vi "Raman Live Tool Set v10.1.0.vi"(1 "Exit":bool, 2 "LiveData":dbl[][](array[numeric]), 3 "RemoteIndicator":bool) -> ()   [LabVIEW 2010]
uses:
  subvi/_TypeDefs/MapFunctions.ctl
  <vilib>/Utility/miscctls.llb/LVPointTypeDef.ctl
  <vilib>/Utility/miscctls.llb/LVStringsAndValuesArrayTypeDef.ctl
  <vilib>/Utility/inputDevices.llb/closeKeyboard.vi
  <vilib>/Utility/inputDevices.llb/keyboardAcquire.vi
  <vilib>/Utility/file.llb/Read From Spreadsheet File (DBL).vi
  <vilib>/Analysis/NI_AALBase.lvlib
panel:
  in  "MapFunction":T1 caption="Mapping function" items=["Total"=0, "Peak"=4, "Area"=2, "Value"=1, "Ratio"=3]
  in  "CreateMap":bool
  in  "SpectrumCoerce":dbl caption="Limit?"
  out "XY Full Interpol.":cluster{dbl, dbl}[](array[cluster])
  out "Axes":T2
  in  "SpectrumNoise":dbl caption="Noise?"
  in  "SpectrumX":u16(ring) caption="X"
  in  "SpectrumY":u16(ring) caption="Y"
  out "Spectrum":cluster{dbl[], dbl[]}(graph) caption="Current Spectrum"
  in  "MapKeyboard":bool
  in  "MapEditColor":bool caption="Edit Color"
  in  "MapFlipColor":bool caption="Flip Color"
  in  "MapInterpolate":bool
  in  "MapSaveData":bool
  out "Map":dbl[][](graph)
  out "LoadingSpectra":bool
  in  "SourceFile":path caption="Mapping File"
  in  "MapCursorDummy":bool
  out "XY Unique":cluster{"X Unique":dbl[], "Y Unique":dbl[]}
  out "XY Full":cluster{dbl, dbl}[](array[cluster])
  out "Intensities (2D)":dbl[][](array[numeric])
  out "Wavelengths (1D)":dbl[](array[numeric])
  out "MapColorTable":u32[](array[numeric])=[0, 196608, 393216, 589824, 786432, 983040, 1179648, 1376256, 1572864, 1769472, 1966080, 2162688, 2359296, 2555904, 2752512, 2949120, 3145728, 3342336, 3538944, 3735552, 3932160, 4128768, 4325376, 4521984, 4718592, 4915200, 5111808, 5308416, 5505024, 5701632, 5898240, 6094848, 6291456, 6488064, 6684672, 6881280, 7077888, 7274496, 7471104, 7667712, 7864320, 8060928, 8257536, 8454144, 8650752, 8847360, 9043968, 9240576, 9437184, 9633792, 9830400, 10027008, 10223616, 10420224, 10616832, 10813440, 11010048, 11206656, 11403264, 11599872, 11796480, 11993088, 12189696, 12386304, 12582912, 12779520, 12976128, 13172736, 13369344, 13565952, 13762560, 13959168, 14155776, 14352384, 14548992, 14745600, 14942208, 15138816, 15335424, 15532032, 15728640, 15925248, 16121856, 16318464, 16515072, 16711680, 16712448, 16713216, 16713984, 16714752, 16715520, 16716288, 16717056, 16717824, 16718592, 16719360, 16720128, 16720896, 16721664, 16722432, 16723200, 16723968, 16724736, 16725504, 16726272, 16727040, 16727808, 16728576, 16729344, 16730112, 16730880, 16731648, 16732416, 16733184, 16733952, 16734720, 16735488, 16736256, 16737024, 16737792, 16738560, 16739328, 16740096, 16740864, 16741632, 16742400, 16743168, 16743936, 16744704, 16745472, 16746240, 16747008, 16747776, 16748544, 16749312, 16750080, 16750848, 16751616, 16752384, 16753152, 16753920, 16754688, 16755456, 16756224, 16756992, 16757760, 16758528, 16759296, 16760064, 16760832, 16761600, 16762368, 16763136, 16763904, 16764672, 16765440, 16766208, 16766976, 16767744, 16768512, 16769280, 16770048, 16770816, 16771584, 16772352, 16773120, 16773888, 16774656, 16775424, 16776192, 16776960, 16776963, 16776966, 16776969, 16776972, 16776975, 16776977, 16776980, 16776983, 16776986, 16776989, 16776992, 16776995, 16776998, 16777001, 16777004, 16777007, 16777009, 16777012, 16777015, 16777018, 16777021, 16777024, 16777027, 16777030, 16777033, 16777036, 16777038, 16777041, 16777044, 16777047, 16777050, 16777053, 16777056, 16777059, 16777062, 16777065, 16777068, 16777070, 16777073, 16777076, 16777079, 16777082, 16777085, 16777088, 16777091, 16777094, 16777097, 16777100, 16777102, 16777105, 16777108, 16777111, 16777114, 16777117, 16777120, 16777123, 16777126, 16777129, 16777132, 16777134, 16777137, 16777140, 16777143, 16777146, 16777149, 16777152, 16777155, 16777158, 16777161, 16777163, 16777166, 16777169, 16777172, 16777175, 16777178, 16777181, 16777184, 16777187, 16777190, 16777193, 16777195, 16777198, 16777201, 16777204, 16777207]
  out "MapZBounds":cluster{dbl, dbl}
  out "MapData (2D)":dbl[][](array[numeric])
  # "Cursor"
  # "Map Function"
  # "Spectrum"
  # "Raman Live Tool Set"
  # "by A. Schmitz-Wunderlich, P. Candeloro"
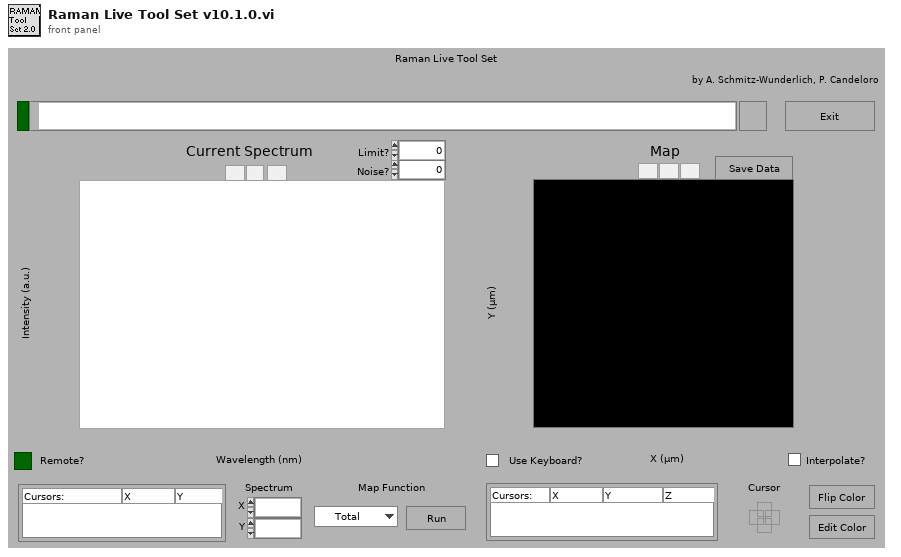
[diagram p1: front panel]
types:
  T1 = typedef "MapFunctions.ctl" = u16
  T2 = cluster{"X":cluster{"Offset":dbl, "Step Size":dbl, "Step Count":i32}, "Y":cluster{"Offset":dbl, "Step Size":dbl, "Step Count":i32}}
  T3 = typedef "LVPointTypeDef.ctl" = cluster{"Horizontal":i16, "Vertical":i16}
  T4 = enum8{"Enabled", "Disabled", "Disabled and Grayed Out"}
  T5 = enum16{"0", "1", "2", "3", "4", "5", "6", "7", "8", "9", "A", "B", "C", "D", "E", "F", "G", "H", "I", "J", "K", "L", "M", "N", "O", "P", "Q", "R", "S", "T", "U", "V", "W", "X", "Y", "Z", "F1", "F2", "F3", "F4", "F5", "F6", "F7", "F8", "F9", "F10", "F11", "F12", "F13", "F14", "F15", "ADD", "BACK", "BACKSLASH", "CAPITAL", "COMMA", "DECIMAL", "DELETE", "DIVIDE", "DOWN", "END", "EQUALS", "ESCAPE", "GRAVE (`)", "HOME", "INSERT", "LBRACKET", "LCONTROL", "LEFT", "L ALT", "LSHIFT", "LWIN", "MINUS", "MULTIPLY", "NEXT", "NUMLOCK", "NUMPAD_0", "NUMPAD_1", "NUMPAD_2", "NUMPAD_3", "NUMPAD_4", "NUMPAD_5", "NUMPAD_6", "NUMPAD_7", "NUMPAD_8", "NUMPAD_9", "PAUSE", "PERIOD", "PRIOR (PG UP)", "RBRACKET", "RCONTROL", "RETURN", "RIGHT", "R ALT", "RSHIFT", "RWIN", "SCROLL", "SEMICOLON", "SLASH", "SPACE", "SUBTRACT", "TAB", "UP", "ENTER (num pad)", "' (quote)"}
  T6 = enum16{"0", "1", "2", "3", "4", "5", "6", "7", "8", "9", "A", "B", "C", "D", "E", "F", "G", "H", "I", "J", "K", "L", "M", "N", "O", "P", "Q", "R", "S", "T", "U", "V", "W", "X", "Y", "Z", "F1", "F2", "F3", "F4", "F5", "F6", "F7", "F8", "F9", "F10", "F11", "F12", "F13", "F14", "F15", "ADD", "BACK", "BACKSLASH", "CAPITAL", "COMMA", "DECIMAL", "DELETE", "DIVIDE", "DOWN", "END", "EQUALS", "ESCAPE", "GRAVE (`)", "HOME", "INSERT", "LBRACKET", "LCONTROL", "LEFT", "L ALT", "LSHIFT", "LWIN", "MINUS", "MULTIPLY", "NEXT", "NUMLOCK", "NUMPAD_0", "NUMPAD_1", "NUMPAD_2", "NUMPAD_3", "NUMPAD_4", "NUMPAD_5", "NUMPAD_6", "NUMPAD_7", "NUMPAD_8", "NUMPAD_9", "PAUSE", "PERIOD", "PRIOR (PG UP)", "RBRACKET", "RCONTROL", "RETURN", "RIGHT", "R ALT", "RSHIFT", "RWIN", "SCROLL", "SEMICOLON", "SLASH", "SPACE", "SUBTRACT", "TAB", "UP", "ENTER (num pad)", "' (quote)"}[]
  T7 = cluster{"Name":string, "Color":u32, "Style":u8, "Point Style":u8, "Name Visible":bool, "Allow Drag":bool, "Cursor Mode":u32, "Plot":i32, "Index":i32, "Position":cluster{"X":dbl, "Y":dbl}, "X Scale":u32, "Y Scale":u32, "Watch Plots":i32[], "Watch All Plots":bool, "Plot Area":i32, "Label Offset":cluster{"X":dbl, "Y":dbl}}
  T8 = cluster{"Name":string, "Color":u32, "Style":u8, "Point Style":u8, "Name Visible":bool, "Allow Drag":bool, "Cursor Mode":u32, "Plot":i32, "Index":i32, "Position":cluster{"X":dbl, "Y":dbl}, "X Scale":u32, "Y Scale":u32, "Watch Plots":i32[], "Watch All Plots":bool, "Plot Area":i32, "Label Offset":cluster{"X":dbl, "Y":dbl}}[]
  T9 = typedef "LVCursorListTypeDef.ctl" = cluster{"Name":string, "Color":u32, "Style":u8, "Point Style":u8, "Name Visible":bool, "Allow Drag":bool, "Cursor Mode":u32, "Plot":i32, "Index":i32, "Position":cluster{"X":dbl, "Y":dbl}, "X Scale":u32, "Y Scale":u32, "Watch Plots":i32[], "Watch All Plots":bool, "Plot Area":i32, "Label Offset":cluster{"X":dbl, "Y":dbl}}[]
  T10 = typedef "LVPointDoubleTypeDef.ctl" = cluster{"Cursor X":dbl, "Cursor Y":dbl}
  T11 = typedef "LVStringsAndValuesArrayTypeDef.ctl" = cluster{"String":string, "Value":ext}[]
  T12 = enum32{"invalid app kind", "Development System", "Run Time System", "Student Edition", "Embedded LabVIEW", "Evaluation", "Custom"}
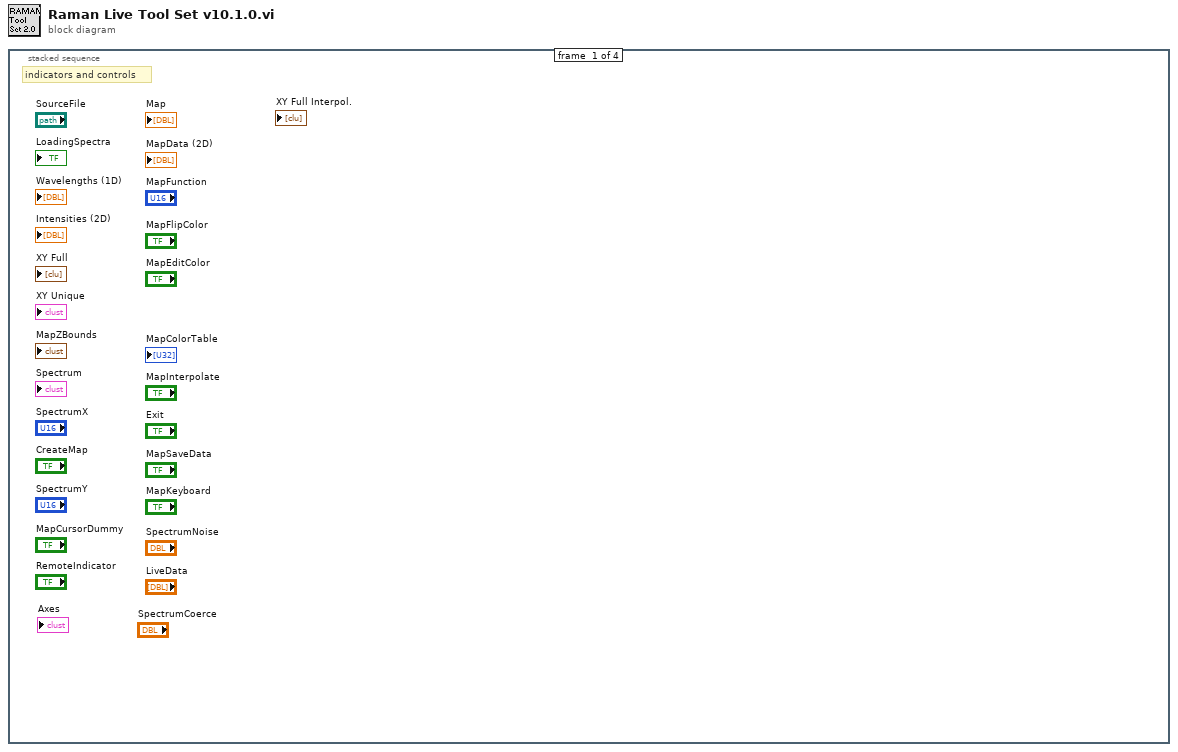
[diagram p0: block diagram]
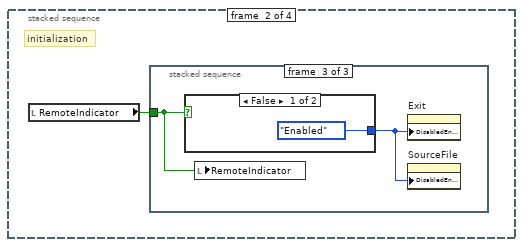
[diagram p2: hidden frame]
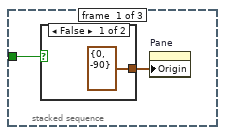
[diagram p3: hidden frame]
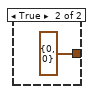
[diagram p4: hidden frame]
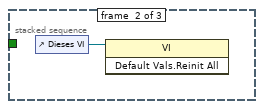
[diagram p5: hidden frame]
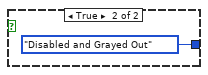
[diagram p6: hidden frame]
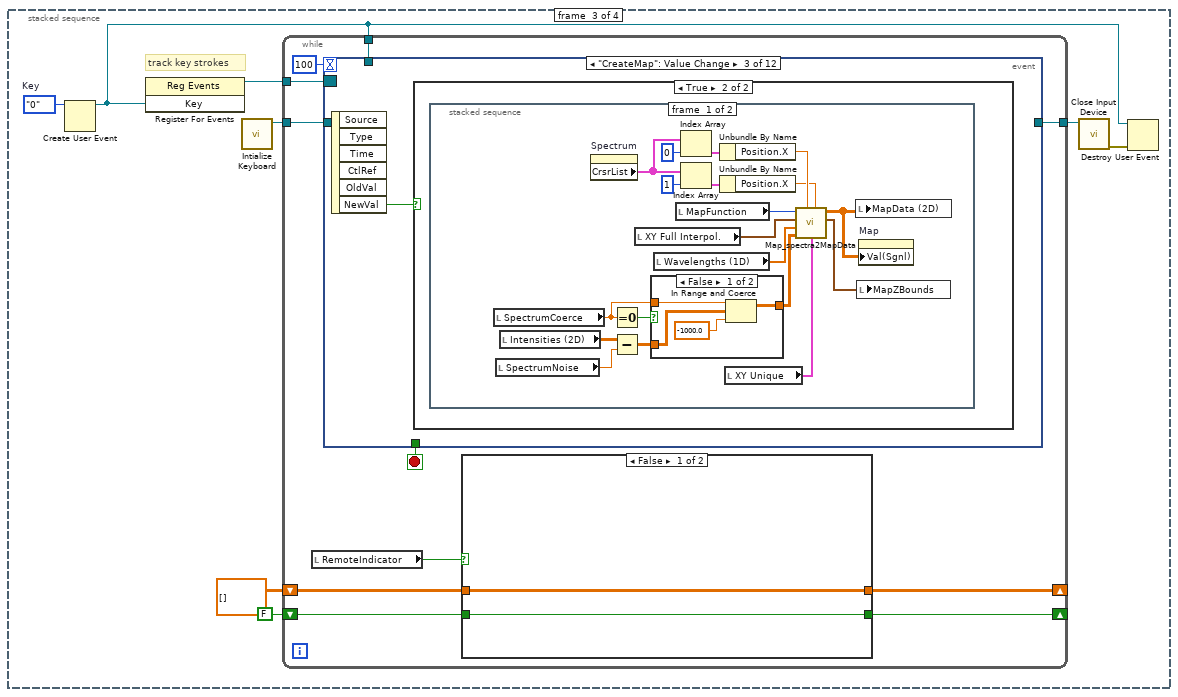
[diagram p7: hidden frame]
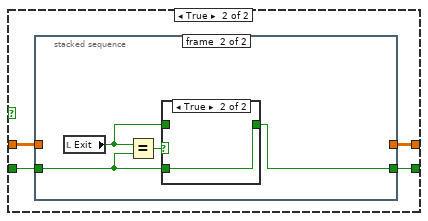
[diagram p8: hidden frame]
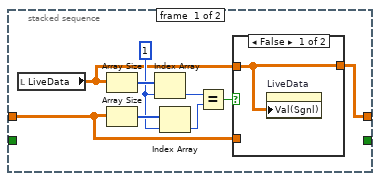
[diagram p9: hidden frame]
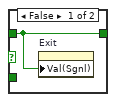
[diagram p11: hidden frame]
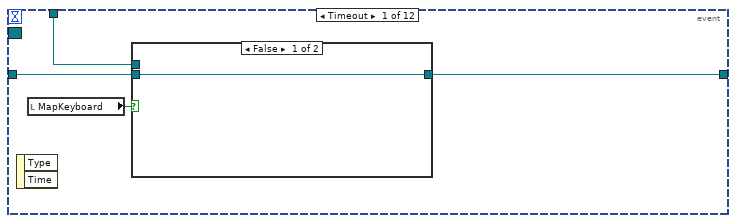
[diagram p12: hidden frame]
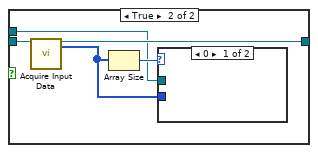
[diagram p13: hidden frame]
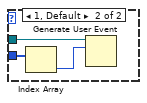
[diagram p14: hidden frame]
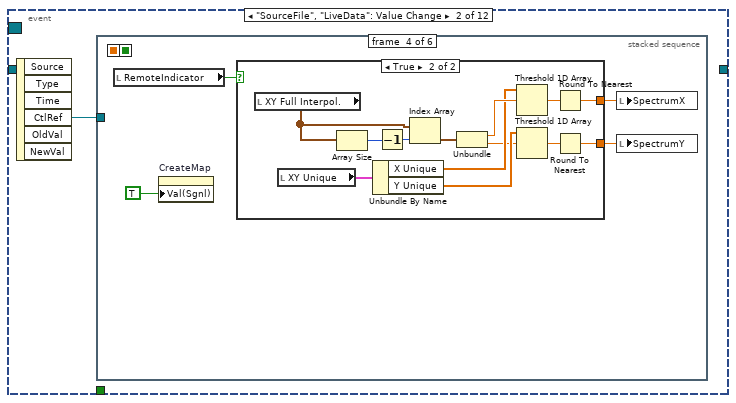
[diagram p15: hidden frame]
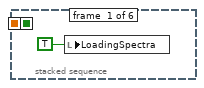
[diagram p16: hidden frame]
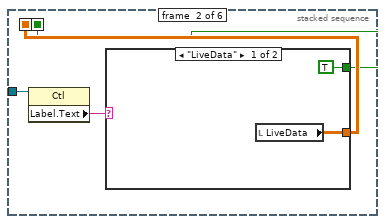
[diagram p17: hidden frame]
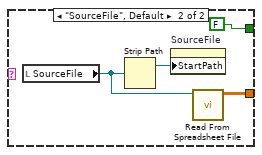
[diagram p18: hidden frame]
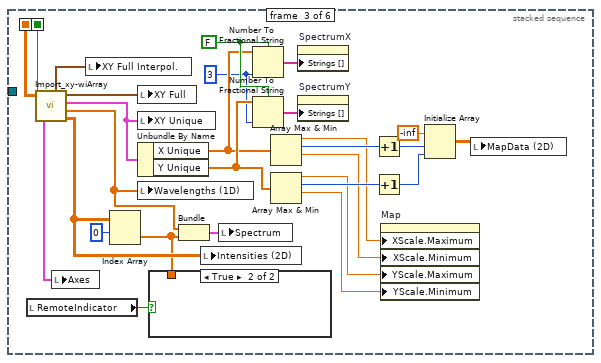
[diagram p19: hidden frame]
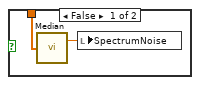
[diagram p20: hidden frame]
diagram:
  n1 = stacked-sequence {
    frame #0 {
      # "indicators and controls"
    }
    frame #1 {
      # "initialization"
      n2 = local read "RemoteIndicator"() -> (w1:bool)
      n3 = stacked-sequence {
        tunnel: w1 -> [w2 _ w7]
        frame #0 {
          n4 = case shown="False" w2 {
            tunnel: [T3 {"Horizontal"=0, "Vertical"=-90} ("Origin") T3 {"Horizontal"=0, "Vertical"=0} ("Origin")] -> w3
            frame False {
            }
            frame True {
            }
          }
          n5 = property on="Pane" class="Pane"("Origin"=w3) -> ()  [unwired: 2 in, 2 out]
        }
        frame #1 {
          n6 = control-ref of="Dieses VI"() -> (w6:refnum<vi>)
          n7 = invoke class="VI" method="Default Vals.Reinit All"(reference=w6) -> ()  [unwired: 2 in, 3 out]
        }
        frame #2 {
          n8 = case shown="False" w7 {
            tunnel: [T4."Enabled" ("Deaktiviert") T4."Disabled and Grayed Out" ("Deaktiviert")] -> w8
            frame False {
            }
            frame True {
            }
          }
          n9 = local write "RemoteIndicator"(w7) -> ()
          n10 = property on="Exit" class="Bool (strict)"("DisabledEnum"=w8) -> ()  [unwired: 2 in, 2 out]
          n11 = property on="SourceFile" class="Path"("DisabledEnum"=w8) -> ()  [unwired: 2 in, 2 out]
        }
      }
    }
    frame #2 {
      w18 = T5."0"  # Key
      # "track key strokes"
      n12 = Create User Event(user event datatype=w18) -> (user event=w15:refnum<user-event>)  [unwired: 1 in, 1 out]
      n13 = register-events(w15) -> (reference out=w16:refnum<event-registration>)  [unwired: 2 in, 1 out]
      n14 = call <vilib>:"Intialize Keyboard.vi"() -> ("device ID"=w14:refnum<k1>)  [unwired: 10 in, 1 out]
      n15 = while {
        tunnel: w16 -> [w28]
        tunnel: w15 -> [w27]
        tunnel: w14 -> [w26]
        tunnel: [w25] -> w13
        shift-right: [w21] -> _
        shift-left: dbl[][] [] ("LiveData") -> [w22]
        shift-right: [w19] -> _
        shift-left: FALSE -> [w20]
        stop <- w29 stop-if-true
        n16 = local read "RemoteIndicator"() -> (w23:bool)
        n17 = event shown="[2] \"CreateMap\": Value Change" {
          selector: w28 -> [_ _ _ _ _ _ _ _ _ _ _ _]
          dyn-events: _ -> [_ _ _ _ _ _ _ _ _ _ _ _]
          timeout: 100 -> [_ _ _ _ _ _ _ _ _ _ _ _]
          tunnel: [_ _ _ _ _ _ _ _ _ _ _ w329] -> w29
          tunnel: w27 -> [w56 _ _ _ _ _ _ _ _ _ _ _]
          tunnel: w26 -> [w55 _ _ _ _ _ _ _ _ _ _ _]
          tunnel: [w53 _ _ _ _ _ _ _ _ _ _ _] -> w25
          event Timeout {
            n18 = event-data() -> ()  [unwired: 1 in, 2 out]
            n19 = local read "MapKeyboard"() -> (w54:bool)
            n20 = case shown="False" w54 {
              tunnel: [w57 w62] -> w53
              tunnel: w56 -> [_ w59]
              tunnel: w55 -> [w57 w58]
              frame False {
              }
              frame True {
                n21 = call-poly <vilib>:"Acquire Input Data.vi"("device ID"=w58) -> ("device ID"=w62:refnum<k1>, "keys pressed"=w61:T6)  [unwired: 16 in, 1 out]
                n22 = Array Size(array=w61) -> (size(s)=w60:i32)
                n23 = case shown="0" w60 {
                  tunnel: w59 -> [_ w65]
                  tunnel: w61 -> [_ w63]
                  frame 0 {
                  }
                  frame 1, Default {
                    n24 = Index Array(array=w63) -> (element=w64:T5)  [unwired: 1 in]
                    n25 = Generate User Event(user event=w65, event data cluster=w64) -> ()  [unwired: 1 in, 2 out]
                  }
                }
              }
            }
          }
          event "SourceFile", "LiveData": Value Change {
            n26 = event-data() -> ("CtlRef"=w66:refnum<vi>)  [unwired: 1 in, 5 out]
            n27 = stacked-sequence {
              seq-local: [_ w69 _ _ _ _] -> [_ _ w87 _ _ _]
              seq-local: [_ w68 _ _ _ _] -> [_ _ w80 _ _ _]
              tunnel: w66 -> [_ w71 _ _ _ _]
              frame #0 {
                n28 = local write "LoadingSpectra"(TRUE ("Loading\nSpectra")) -> ()
              }
              frame #1 {
                n29 = property class="Ctl"(reference=w71) -> ("Label.Text"=w70:string)  [unwired: 1 in, 2 out]
                n30 = case shown="\"LiveData\"" w70 {
                  tunnel: [w73 w75] -> w69
                  tunnel: [TRUE FALSE] -> w68
                  frame "LiveData" {
                    n31 = local read "LiveData"() -> (w73:dbl[][])
                  }
                  frame "SourceFile", Default {
                    n32 = local read "SourceFile"() -> (w76:path)
                    n33 = Strip Path(path=w76) -> (stripped path=w77:path)  [unwired: 1 out]
                    n34 = property on="SourceFile" class="Path"("StartPath"=w77) -> ()  [unwired: 2 in, 2 out]
                    n35 = call-poly <vilib>:"Read From Spreadsheet File.vi"("file path (dialog if empty)"=w76) -> ("all rows"=w75:dbl[][])  [unwired: 6 in, 4 out]
                  }
                }
              }
              frame #2 {
                w94 = i16 3 ("Genauigkeit (6)")
                w101 = FALSE ("Systemdezimalzeichen verwenden (T)")
                n36 = local read "RemoteIndicator"() -> (w81:bool)
                n37 = call "Import_xy-wiArray.vi"("InputArray"=w87, "Uniform"=w80) -> ("XY Full"=w79:cluster{dbl, dbl}[], "XY Unique"=w84:cluster{"X Unique":dbl[], "Y Unique":dbl[]}, "Wavelength"=w85:dbl[], "Intensity"=w86:dbl[][], "XY Full Interpol."=w78:cluster{dbl, dbl}[], "Axes"=w82:T2)
                n38 = local write "Axes"(w82) -> ()
                n39 = local write "XY Full Interpol."(w78) -> ()
                n40 = Index Array(array=w86, index (row)=0 ("Index (Zeile)")) -> (element=w83:dbl[])  [unwired: 1 in]
                n41 = local write "XY Full"(w79) -> ()
                n42 = local write "XY Unique"(w84) -> ()
                n43 = Unbundle By Name(w84) -> ("X Unique"=w95:dbl[], "Y Unique"=w96:dbl[])
                n44 = local write "Wavelengths (1D)"(w85) -> ()
                n45 = case shown="True" w81 {
                  tunnel: w83 -> [w106 _]
                  frame False {
                    n46 = call <vilib>:"Median.vi"("X"=w106) -> ("median"=w107:dbl)  [unwired: 1 out]
                    n47 = local write "SpectrumNoise"(w107) -> ()
                  }
                  frame True {
                  }
                }
                n48 = Bundle("Wavelength"=w85, "Intensity"=w83) -> (w105:cluster{"Wavelength":dbl[], "Intensity":dbl[]})  [unwired: 1 in]
                n49 = local write "Intensities (2D)"(w86) -> ()
                n50 = local write "Spectrum"(w105) -> ()
                n51 = Number To Fractional String(use system decimal point (T)=w101, number=w95, precision (6)=w94) -> (F-format string=w98:string[])  [unwired: 1 in]
                n52 = Number To Fractional String(use system decimal point (T)=w101, number=w96, precision (6)=w94) -> (F-format string=w97:string[])  [unwired: 1 in]
                n53 = Array Max & Min(array=w95) -> (max value=w91:dbl, max index (indices)=w93:i32, min value=w90:dbl)  [unwired: 1 out]
                n54 = Array Max & Min(array=w96) -> (max value=w89:dbl, max index (indices)=w92:i32, min value=w88:dbl)  [unwired: 1 out]
                n55 = property on="SpectrumX" class="Ring (strict)"("Strings []"=w98) -> ()  [unwired: 2 in, 2 out]
                n56 = property on="SpectrumY" class="Ring (strict)"("Strings []"=w97) -> ()  [unwired: 2 in, 2 out]
                n57 = Increment(x=w93) -> (x+1=w102:i32)
                n58 = Increment(x=w92) -> (x+1=w103:i32)
                n59 = property on="Map" class="IntGraph (strict)"("XScale.Maximum"=w91, "XScale.Minimum"=w90, "YScale.Maximum"=w89, "YScale.Minimum"=w88) -> ()  [unwired: 2 in, 2 out]
                n60 = Initialize Array(-inf, w102, w103) -> (w100:dbl[][])
                n61 = local write "MapData (2D)"(w100) -> ()
              }
              frame #3 {
                n62 = local read "RemoteIndicator"() -> (w111:bool)
                n63 = property on="CreateMap" class="Bool (strict)"("Val(Sgnl)"=TRUE ("Wert (signalisierend)")) -> ()  [unwired: 2 in, 2 out]
                n64 = case shown="True" w111 {
                  tunnel: [w112 w113] -> w110
                  tunnel: [w112 w114] -> w109
                  frame False {
                    w112 = 0
                  }
                  frame True {
                    n65 = local read "XY Full Interpol."() -> (w122:cluster{dbl, dbl}[])
                    n66 = local read "XY Unique"() -> (w125:cluster{"X Unique":dbl[], "Y Unique":dbl[]})
                    n67 = Array Size(array=w122) -> (size(s)=w124:i32)
                    n68 = Unbundle By Name(w125) -> ("X Unique"=w118:dbl[], "Y Unique"=w117:dbl[])
                    n69 = Decrement(x=w124) -> (x-1=w123:i32)
                    n70 = Index Array(array=w122, index=w123) -> (element=w121:cluster{dbl, dbl})
                    n71 = Unbundle(w121) -> (w119:dbl, w116:dbl)
                    n72 = Threshold 1D Array(2:w119, 3:w118) -> (0:w120:dbl)  [unwired: 1 in]
                    n73 = Threshold 1D Array(2:w116, 3:w117) -> (0:w115:dbl)  [unwired: 1 in]
                    n74 = Round To Nearest(number=w120) -> (nearest integer value=w113:dbl)
                    n75 = Round To Nearest(number=w115) -> (nearest integer value=w114:dbl)
                  }
                }
                n76 = local write "SpectrumX"(w110) -> ()
                n77 = local write "SpectrumY"(w109) -> ()
              }
              frame #4 {
                w135 = i8 2 ("y")
                w143 = T7 {"Name"="cursor", "Color"=1985280, "Style"=2, "Point Style"=6, "Name Visible"=FALSE, "Allow Drag"=TRUE, "Cursor Mode"=0, "Plot"=0, "Index"=0, "Position"={"X"=0.0, "Y"=0.0}, "X Scale"=0, "Y Scale"=0, "Watch Plots"=[], "Watch All Plots"=FALSE, "Plot Area"=0, "Label Offset"={"X"=0.0, "Y"=0.0}}  # cursorConst
                n78 = local read "Axes"() -> (w139:T2)
                n79 = Unbundle By Name(w139) -> ("X.Offset"=w138:dbl, "X.Step Size"=w137:dbl, "Y.Offset"=w134:dbl, "Y.Step Size"=w136:dbl)
                n80 = Divide(x=w137, y=w135) -> (x/y=w133:dbl)
                n81 = Divide(x=w136, y=w135) -> (x/y=w132:dbl)
                n82 = Add(x=w138, y=w133) -> (x+y=w130:dbl)
                n83 = Add(x=w134, y=w132) -> (x+y=w131:dbl)
                n84 = Bundle(w130, w131) -> (w128:cluster{dbl, dbl})  [unwired: 1 in]
                n85 = Bundle By Name(cluster=w143, "Name"="Spot", "Cursor Mode"=u32 0, "Position"=w128) -> (w127:T7)
                n86 = Build Array(w127) -> (w126:T8)
                n87 = property on="Map" class="IntGraph (strict)"("CrsrLis"=w126, "Cursor.Cursor Style"=u8 8, "Cursor.Cursor Point Style"=u8 5, "Cursor.Cursor Color"=u32 16448250 ("Color")) -> ()  [unwired: 2 in, 2 out]
              }
              frame #5 {
                n88 = local write "LoadingSpectra"(FALSE ("Loading\nSpectra")) -> ()
              }
            }
          }
          event "CreateMap": Value Change {
            n89 = event-data() -> ("NewVal"=w146:bool)  [unwired: 1 in, 5 out]
            n90 = case shown="True" w146 {
              frame False {
              }
              frame True {
                n91 = stacked-sequence {
                  frame #0 {
                    n92 = local read "SpectrumCoerce"() -> (w151:dbl)
                    n93 = local read "SpectrumNoise"() -> (w154:dbl)
                    n94 = local read "Intensities (2D)"() -> (w147:dbl[][])
                    n95 = property on="Spectrum" class="XYGraph (strict)"() -> ("CrsrList"=w158:T9)  [unwired: 2 in, 2 out]
                    n96 = Equal To 0?(x=w151) -> (x = 0?=w150:bool)
                    n97 = Subtract(x=w147, y=w154) -> (x-y=w148:dbl[][])
                    n98 = local read "XY Full Interpol."() -> (w153:cluster{dbl, dbl}[])
                    n99 = case shown="False" w150 {
                      tunnel: w151 -> [w169 _]
                      tunnel: [w168 w170] -> w149
                      tunnel: w148 -> [w167 w170]
                      frame False {
                        n100 = In Range and Coerce(upper limit=w169, x=w167, lower limit=-1000.0 ("SpectrumCoerce")) -> (coerced(x)=w168:dbl[][])  [unwired: 1 out]
                      }
                      frame True {
                      }
                    }
                    n101 = local read "Wavelengths (1D)"() -> (w165:dbl[])
                    n102 = local read "MapFunction"() -> (w155:T1)
                    n103 = Index Array(array=w158, index=0 ("Index")) -> (element=w161:T7)
                    n104 = Index Array(array=w158, index=1 ("Index")) -> (element=w162:T7)
                    n105 = Unbundle By Name(w161) -> ("Position.X"=w157:dbl)
                    n106 = Unbundle By Name(w162) -> ("Position.X"=w156:dbl)
                    n107 = local read "XY Unique"() -> (w152:cluster{"X Unique":dbl[], "Y Unique":dbl[]})
                    n108 = call "Map_spectra2MapData.vi"("Intensity"=w149, "Wavelength"=w165, "XY Unique"=w152, "XY Full"=w153, "MapFunction"=w155, "X1"=w157, "X2"=w156) -> ("MapZBounds"=w163:cluster{sgl, sgl}, "MapData"=w164:sgl[][])  [unwired: 2 in]
                    n109 = local write "MapData (2D)"(w164) -> ()
                    n110 = local write "MapZBounds"(w163) -> ()
                    n111 = property on="Map" class="IntGraph (strict)"("Val(Sgnl)"=w164) -> ()  [unwired: 2 in, 2 out]
                  }
                  frame #1 {
                    n112 = local read "SpectrumX"() -> (w172:u16)
                    n113 = local write "CreateMap"(FALSE ("Value")) -> ()
                    n114 = property on="SpectrumX" class="Ring (strict)"("Val(Sgnl)"=w172) -> ()  [unwired: 2 in, 2 out]
                  }
                }
              }
            }
          }
          event "Map", "MapInterpolate", "MapFlipColor": Value Change {
            n115 = event-data() -> ()  [unwired: 1 in, 6 out]
            n116 = stacked-sequence {
              seq-local: [w173 _ _ _ _] -> [_ _ w198 _ _]
              frame #0 {
                n117 = local read "MapInterpolate"() -> (w178:bool)
                n118 = local read "MapData (2D)"() -> (w177:dbl[][])
                n119 = local read "XY Unique"() -> (w174:cluster{"X Unique":dbl[], "Y Unique":dbl[]})
                n120 = local read "Axes"() -> (w176:T2)
                n121 = case shown="True" w178 {
                  tunnel: [w180 w184] -> w175
                  tunnel: w177 -> [w180 w185]
                  tunnel: w176 -> [w179 _]
                  tunnel: w174 -> [_ w182]
                  tunnel: [w179 w181] -> w173
                  frame False {
                  }
                  frame True {
                    n122 = call "Map_interpolateXYZ.vi"("Level"=3, "MapData (2D)"=w185, "XY Unique"=w182) -> ("Z Interpoliert"=w184:dbl[][], "Axes"=w181:T2)  [unwired: 1 out]
                  }
                }
                n123 = local write "Map"(w175) -> ()
              }
              frame #1 {
                w193 = u32 0 ("Color")
                n124 = local read "MapColorTable"() -> (w191:u32[])
                n125 = local read "MapZBounds"() -> (w192:cluster{dbl, dbl})
                n126 = local read "MapFlipColor"() -> (w190:bool)
                n127 = Unbundle(w192) -> (w196:dbl, w189:dbl)
                n128 = Greater Than 0?(x=w189) -> (x > 0?=w187:bool)
                n129 = Reverse 1D Array(array=w191) -> (reversed array=w195:u32[])
                n130 = Select(t=w189, s=w187, f=0.0) -> (s? t:f=w186:dbl)
                n131 = Select(t=w195, s=w190, f=w191) -> (s? t:f=w194:u32[])
                n132 = property on="Map" class="IntGraph (strict)"("ZScale.Interpolate Color"=TRUE ("Z Scale.Interpolate Color"), "ZScale.Maximum"=w196, "ZScale.Minimum"=w186, "Color Table"=w194, "ZScale.High Color"=w193, "ZScale.Low Color"=w193) -> ()  [unwired: 2 in, 2 out]
              }
              frame #2 {
                n133 = Unbundle By Name(w198) -> ("X.Offset"=w202:dbl, "X.Step Size"=w201:dbl, "Y.Offset"=w200:dbl, "Y.Step Size"=w199:dbl)
                n134 = property on="Map" class="IntGraph (strict)"("XScale.Offset"=w202, "XScale.Multiplier"=w201, "YScale.Offset"=w200, "YScale.Multiplier"=w199) -> ()  [unwired: 2 in, 2 out]
              }
              frame #3 {
                w203 = u8 1 ("X-Achse.Achsenanpassung")
                n135 = property on="Map" class="IntGraph (strict)"("XScale.ScaleFit"=w203, "YScale.ScaleFit"=w203, "ZScale.ScaleFit"=u8 0 ("Z-Achse.Achsenanpassung")) -> ()  [unwired: 2 in, 2 out]
              }
              frame #4 {
                n136 = local read "SpectrumX"() -> (w205:u16)
                n137 = property on="SpectrumX" class="Ring (strict)"("Val(Sgnl)"=w205) -> ()  [unwired: 2 in, 2 out]
              }
            }
          }
          event "MapEditColor": Value Change {
            n138 = event-data() -> ("NewVal"=w206:bool)  [unwired: 1 in, 5 out]
            n139 = case shown="True" w206 {
              frame False {
              }
              frame True {
                n140 = flat-sequence {
                  frame #0 {
                    n141 = local read "MapColorTable"() -> (w207:u32[])
                    n142 = call "MapColor_makeRamp.vi"("ColorMap\narray IN"=w207) -> ("ColorMap\narray OUT"=w208:u32[])
                    n143 = local write "MapColorTable"(w208) -> ()
                  }
                  frame #1 {
                    n144 = local read "MapData (2D)"() -> (w210:dbl[][])
                    n145 = local write "MapEditColor"(FALSE ("Value")) -> ()
                    n146 = property on="Map" class="IntGraph (strict)"("Val(Sgnl)"=w210) -> ()  [unwired: 2 in, 2 out]
                  }
                }
              }
            }
          }
          event "MapSaveData": Value Change {
            n147 = event-data() -> ("NewVal"=w211:bool)  [unwired: 1 in, 5 out]
            n148 = case shown="True" w211 {
              frame False {
              }
              frame True {
                n149 = flat-sequence {
                  frame #0 {
                    n150 = property on="MapFunction" class="Ring (strict)"() -> ("RingText.Text"=w213:string)  [unwired: 2 in, 2 out]
                    n151 = local read "SourceFile"() -> (w212:path)
                    n152 = control-ref of="Spectrum"() -> (w214:refnum<vi>)
                    n153 = call "Export_mapFileName.vi"("MapFunctionStr"=w213, "Spectrum"=w214, "SourceFile"=w212) -> ("Dateipfad"=w215:path)
                    n154 = local read "XY Full"() -> (w216:cluster{dbl, dbl}[])
                    n155 = local read "Map"() -> (w217:dbl[][])
                    n156 = call "Export_map2Text.vi"("MapData (2D)"=w217, "XY Full"=w216, "ExportPath"=w215) -> ()  [unwired: 1 in]
                  }
                  frame #1 {
                    n157 = local write "MapSaveData"(FALSE ("Value")) -> ()
                    n158 = Wait (ms)(milliseconds to wait=u32 300) -> ()  [unwired: 1 out]
                  }
                }
              }
            }
          }
          event Value Change {
            n159 = event-data() -> ()  [unwired: 1 in, 6 out]
            n160 = local read "MapFunction"() -> (w220:T1)
            n161 = control-ref of="Spectrum"() -> (w221:refnum<vi>)
            n162 = call "SpectrumCursor_init.vi"("MapFunction"=w220, "Spectrum"=w221) -> ()  [unwired: 1 in]
          }
          event "SpectrumY", "SpectrumX", "SpectrumNoise", "SpectrumCoerce": Value Change {
            n163 = event-data() -> ()  [unwired: 1 in, 6 out]
            n164 = local read "XY Unique"() -> (w239:cluster{"X Unique":dbl[], "Y Unique":dbl[]})
            n165 = local read "SpectrumX"() -> (w234:u16)
            n166 = local read "SpectrumY"() -> (w235:u16)
            n167 = Unbundle By Name(w239) -> ("X Unique"=w237:dbl[], "Y Unique"=w236:dbl[])
            n168 = local read "Intensities (2D)"() -> (w241:dbl[][])
            n169 = local read "SpectrumCoerce"() -> (w225:dbl)
            n170 = local read "XY Full Interpol."() -> (w227:cluster{dbl, dbl}[])
            n171 = local read "SpectrumNoise"() -> (w238:dbl)
            n172 = Index Array(array=w237, index=w234) -> (element=w244:dbl)
            n173 = Index Array(array=w236, index=w235) -> (element=w243:dbl)
            n174 = Bundle(cluster=cluster{dbl, dbl} {0.0, 0.0} ("Element"), w244, w243) -> (w230:cluster{dbl, dbl})
            n175 = Equal To 0?(x=w225) -> (x = 0?=w226:bool)
            n176 = property on="Map" class="IntGraph (strict)"("Cursor.Cursor Position"=w230) -> ()  [unwired: 2 in, 2 out]
            n177 = while {
              tunnel: w227 -> [w256] mode=indexing
              tunnel: w230 -> [w257]
              tunnel: [w255] -> w232
              tunnel: [w252] -> w229
              tunnel: w227 -> [w253]
              i -> [w255]
              stop <- w250 stop-if-true
              n178 = Array Size(array=w253) -> (size(s)=w254:i32)
              n179 = Equal?(x=w256, y=w257) -> (x = y?=w252:bool)
              n180 = Greater?(x=w255, y=w254) -> (0:w251:bool)
              n181 = Or(x=w251, y=w252) -> (x .or. y?=w250:bool)
            }
            n182 = local read "Wavelengths (1D)"() -> (w242:dbl[])
            n183 = Select(t=w232, s=w229, f=u8 0) -> (s? t:f=w228:i32)
            n184 = Index Array(array=w241, index (row)=w228) -> (element=w224:dbl[])  [unwired: 1 in]
            n185 = Subtract(x=w224, y=w238) -> (x-y=w223:dbl[])
            n186 = case shown="False" w226 {
              tunnel: w225 -> [w248 _]
              tunnel: w223 -> [w247 w249]
              tunnel: [w246 w249] -> w222
              frame False {
                n187 = In Range and Coerce(upper limit=w248, x=w247, lower limit=-1000.0 ("SpectrumCoerce")) -> (coerced(x)=w246:dbl[])  [unwired: 1 out]
              }
              frame True {
              }
            }
            n188 = Bundle("Wavelengths (1D)"=w242, w222) -> (w240:cluster{"Wavelengths (1D)":dbl[], dbl[]})  [unwired: 1 in]
            n189 = local write "Spectrum"(w240) -> ()
          }
          event "Map": Cursor Release; "MapCursorDummy": Value Change {
            n190 = event-data() -> ()  [unwired: 1 in, 4 out]
            n191 = property on="Map" class="IntGraph (strict)" props=["Cursor", "Cursor Position", "Cursor", "Cursor Position"]() -> ("Cursor.Cursor Position"=w267:T10)  [unwired: 2 in, 3 out]
            n192 = local read "XY Unique"() -> (w272:cluster{"X Unique":dbl[], "Y Unique":dbl[]})
            n193 = Unbundle By Name(w272) -> ("X Unique"=w260:dbl[], "Y Unique"=w261:dbl[])
            n194 = Unbundle By Name(w267) -> ("Cursor X"=w271:dbl, "Cursor Y"=w270:dbl)
            n195 = Threshold 1D Array(2:w271, 3:w260) -> (0:w266:dbl)  [unwired: 1 in]
            n196 = Threshold 1D Array(2:w270, 3:w261) -> (0:w265:dbl)  [unwired: 1 in]
            n197 = Round To Nearest(number=w266) -> (nearest integer value=w268:dbl)
            n198 = Round To Nearest(number=w265) -> (nearest integer value=w269:dbl)
            n199 = To Unsigned Word Integer(number=w268) -> (unsigned 16bit integer=w258:u16)
            n200 = To Unsigned Word Integer(number=w269) -> (unsigned 16bit integer=w259:u16)
            n201 = Not Equal?(x=w258, y=w266) -> (x != y?=w263:bool)
            n202 = Not Equal?(x=w259, y=w265) -> (x != y?=w264:bool)
            n203 = property on="SpectrumX" class="Ring (strict)"("Val(Sgnl)"=w258) -> ()  [unwired: 2 in, 2 out]
            n204 = property on="SpectrumY" class="Ring (strict)"("Val(Sgnl)"=w259) -> ()  [unwired: 2 in, 2 out]
            n205 = Or(x=w263, y=w264) -> (x .or. y?=w262:bool)
            n206 = case shown="True" w262 {
              tunnel: w261 -> [_ w276]
              tunnel: w260 -> [_ w275]
              tunnel: w259 -> [_ w274]
              tunnel: w258 -> [_ w273]
              frame False {
              }
              frame True {
                n207 = Index Array(array=w275, index=w273) -> (element=w278:dbl)
                n208 = Index Array(array=w276, index=w274) -> (element=w279:dbl)
                n209 = Bundle(w278, w279) -> (w277:cluster{dbl, dbl})  [unwired: 1 in]
                n210 = property on="Map" class="IntGraph (strict)"("Cursor.Cursor Position"=w277) -> ()  [unwired: 2 in, 2 out]
              }
            }
          }
          event "Spectrum": Cursor Release {
            n211 = event-data() -> ()  [unwired: 1 in, 9 out]
            n212 = local read "MapFunction"() -> (w280:T1)
            n213 = control-ref of="Spectrum"() -> (w281:refnum<vi>)
            n214 = call "SpectrumCursor_set.vi"("MapFunction"=w280, "Spectrum"=w281) -> ()
          }
          event User Event {
            n215 = event-data() -> ("Key"=w288:T5)  [unwired: 1 in, 4 out]
            n216 = property on="Map" class="IntGraph (strict)"() -> ("Cursor.Cursor Position"=w289:T10)  [unwired: 2 in, 2 out]
            n217 = local read "Axes"() -> (w282:T2)
            n218 = property on="Map" class="IntGraph (strict)"() -> ("XScale.Maximum"=w293:dbl, "YScale.Maximum"=w292:dbl, "XScale.Minimum"=w291:dbl, "YScale.Minimum"=w290:dbl)  [unwired: 2 in, 2 out]
            n219 = Unbundle By Name(w282) -> ("X.Step Size"=w286:dbl, "Y.Step Size"=w285:dbl)
            n220 = Unbundle By Name(w289) -> ("Cursor X"=w294:dbl, "Cursor Y"=w295:dbl)
            n221 = case shown="\"DOWN\"" w288 {
              tunnel: w291 -> [_ w301 _ _ _]
              tunnel: w293 -> [_ _ w308 _ _]
              tunnel: w292 -> [_ _ _ w315 _]
              tunnel: w290 -> [_ _ _ _ w322]
              tunnel: w294 -> [w299 w300 w307 w319 w326]
              tunnel: w295 -> [w298 w305 w312 w314 w321]
              tunnel: [w298 w305 w312 w318 w325] -> w296
              tunnel: [w299 w304 w311 w319 w326] -> w297
              tunnel: w286 -> [_ w303 w310 _ _]
              tunnel: w285 -> [_ _ _ w316 w323]
              frame "0", Default {
              }
              frame "LEFT" {
                n222 = Subtract(x=w300, y=w303) -> (x-y=w302:dbl)
                n223 = Greater Or Equal?(x=w301, y=w302) -> (x >= y?=w306:bool)
                n224 = Select(t=w300, s=w306, f=w302) -> (s? t:f=w304:dbl)
              }
              frame "RIGHT" {
                n225 = Add(x=w307, y=w310) -> (x+y=w309:dbl)
                n226 = Greater Or Equal?(x=w308, y=w309) -> (x >= y?=w313:bool)
                n227 = Select(t=w309, s=w313, f=w307) -> (s? t:f=w311:dbl)
              }
              frame "UP" {
                n228 = Add(x=w314, y=w316) -> (x+y=w317:dbl)
                n229 = Less Or Equal?(x=w315, y=w317) -> (x <= y?=w320:bool)
                n230 = Select(t=w314, s=w320, f=w317) -> (s? t:f=w318:dbl)
              }
              frame "DOWN" {
                n231 = Subtract(x=w321, y=w323) -> (x-y=w324:dbl)
                n232 = Greater Or Equal?(x=w322, y=w324) -> (x >= y?=w327:bool)
                n233 = Select(t=w321, s=w327, f=w324) -> (s? t:f=w325:dbl)
              }
            }
            n234 = Bundle("Cursor X"=w297, "Cursor Y"=w296) -> (w287:cluster{"Cursor X":dbl, "Cursor Y":dbl})  [unwired: 1 in]
            n235 = local read "MapCursorDummy"() -> (w283:bool)
            n236 = property on="Map" class="IntGraph (strict)"("Cursor.Cursor Position"=w287) -> (error out=w284:errorcluster)  [unwired: 2 in, 1 out]
            n237 = property on="MapCursorDummy" class="Bool (strict)"(error in=w284, "Val(Sgnl)"=w283) -> ()  [unwired: 1 in, 2 out]
          }
          event "Exit": Value Change {
            n238 = event-data() -> ("OldVal"=w328:bool, "NewVal"=w329:bool)  [unwired: 1 in, 4 out]
            n239 = local write "Exit"(w328) -> ()
          }
        }
        n240 = case shown="False" w23 {
          tunnel: w22 -> [w31 w35]
          tunnel: [w31 w34] -> w21
          tunnel: w20 -> [w30 w33]
          tunnel: [w30 w32] -> w19
          frame False {
          }
          frame True {
            n241 = stacked-sequence {
              tunnel: w35 -> [w39 _]
              tunnel: [w38 _] -> w34
              tunnel: w33 -> [_ w47]
              tunnel: [_ w49] -> w32
              frame #0 {
                w42 = 1 ("Index")
                n242 = local read "LiveData"() -> (w40:dbl[][])
                n243 = Array Size(array=w40) -> (size(s)=w43:i32[])
                n244 = Array Size(array=w39) -> (size(s)=w44:i32[])
                n245 = Index Array(array=w43, index=w42) -> (element=w37:i32)
                n246 = Index Array(array=w44, index=w42) -> (element=w36:i32)
                n247 = Equal?(x=w37, y=w36) -> (x = y?=w41:bool)
                n248 = case shown="False" w41 {
                  tunnel: [w45 w46] -> w38
                  tunnel: w39 -> [_ w46]
                  tunnel: w40 -> [w45 _]
                  frame False {
                    n249 = property on="LiveData" class="Arr (strict)"("Val(Sgnl)"=w45) -> ()  [unwired: 2 in, 2 out]
                  }
                  frame True {
                  }
                }
              }
              frame #1 {
                n250 = local read "Exit"() -> (w48:bool)
                n251 = Equal?(x=w48, y=w47) -> (x = y?=w50:bool)
                n252 = case shown="True" w50 {
                  tunnel: [w51 w52] -> w49
                  tunnel: w47 -> [_ w52]
                  tunnel: w48 -> [w51 _]
                  frame False {
                    n253 = property on="Exit" class="Bool (strict)"("Val(Sgnl)"=w51) -> ()  [unwired: 2 in, 2 out]
                  }
                  frame True {
                  }
                }
              }
            }
          }
        }
      }
      n254 = call-poly <vilib>:"Close Input Device.vi"("device ID"=w13) -> ("error out"=w17:errorcluster)  [unwired: 9 in]
      n255 = Destroy User Event(user event=w15, error in=w17) -> ()  [unwired: 1 out]
    }
    frame #3 {
      w332 = T4."Enabled" ("Deaktiviert")
      w333 = T11 [] ("Strings und Werte []")
      w334 = T8 [] ("Cursor List")
      # "reset and shutdown"
      n256 = control-ref of="Dieses VI"() -> (w335:refnum<vi>)
      n257 = invoke class="VI" method="Default Vals.Reinit All"(reference=w335) -> (reference out=w330:refnum<vi>)  [unwired: 2 in, 2 out]
      n258 = property on="SpectrumY" class="Ring (strict)"("StringsAndValues[]"=w333) -> ()  [unwired: 2 in, 2 out]
      n259 = property on="SpectrumX" class="Ring (strict)"("StringsAndValues[]"=w333) -> ()  [unwired: 2 in, 2 out]
      n260 = property on="SourceFile" class="Path"("DisabledEnum"=w332) -> ()  [unwired: 2 in, 2 out]
      n261 = property on="Exit" class="Bool (strict)"("DisabledEnum"=w332) -> ()  [unwired: 2 in, 2 out]
      n262 = property on="Map" class="IntGraph (strict)"("CrsrLis"=w334) -> ()  [unwired: 2 in, 2 out]
      n263 = property on="Spectrum" class="XYGraph (strict)"("CrsrList"=w334) -> ()  [unwired: 2 in, 2 out]
      n264 = property class="App"() -> ("App.Kind"=w331:T12)  [unwired: 2 in, 2 out]
      n265 = case shown="\"Development System\"" w331 {
        tunnel: w330 -> [w336 _]
        frame "invalid app kind", Default {
          n266 = invoke on="Invoke Node" class="VI" method="FP.Close"(reference=w336) -> ()  [unwired: 2 in, 3 out]
        }
        frame "Development System" {
        }
      }
    }
  }
